vi "TCPServerListenLoop.vi"   [LabVIEW 2019]
uses:
  02 Mode/TCPServerMode/TCPServerClass.lvclass
types:
  T1 = typedef "队列枚举.ctl" = enum16{"ini", "读", "写"}
  T2 = map{string, refnum<class "TCPServerClass.lvclass">}
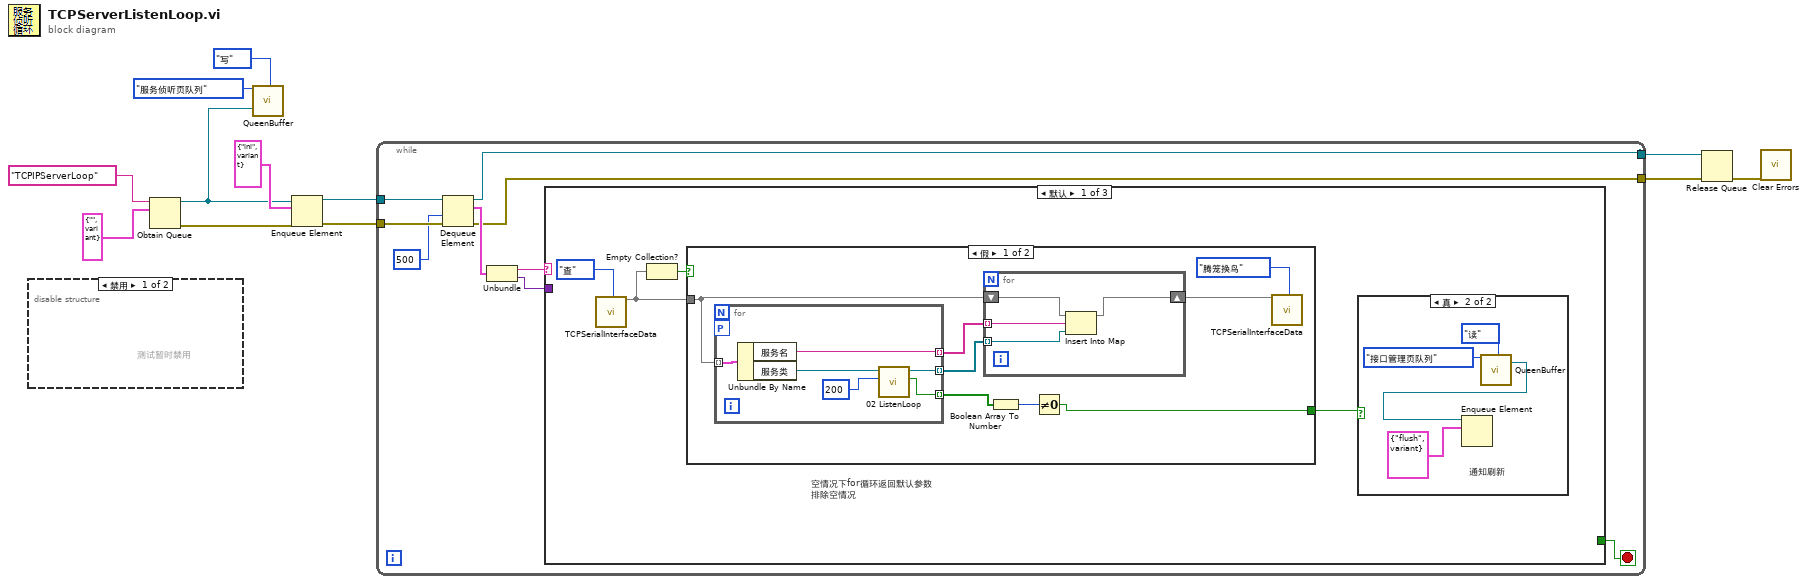
[diagram p0: block diagram]
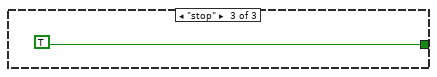
[diagram p6: hidden frame]
diagram:
  n1 = disable-structure shown="禁用" {
    frame Disabled {
      # "测试暂时禁用"
    }
    frame Enabled {
    }
  }
  n2 = Obtain Queue(name (unnamed)="TCPIPServerLoop" ("名称（未命名）"), element data type=cluster{string, variant} {"", variant}) -> (queue out=w1:refnum<queue>, error out=w4:errorcluster)  [unwired: 3 in, 1 out]
  n3 = call "QueenBuffer.vi"("名称"=enum16{"接口管理页队列", "服务侦听页队列", "主页队列"}."服务侦听页队列", "目标队列输入"=w1, "操作"=队列枚举."写") -> ()  [unwired: 16 in, 1 out]
  n4 = Enqueue Element(queue=w1, element=cluster{string, variant} {"ini", variant} ("元素"), error in (no error)=w4) -> (queue out=w11:refnum<queue>, error out=w10:errorcluster)  [unwired: 1 in, 1 out]
  n5 = while {
    tunnel: w11 -> [w21]
    tunnel: w10 -> [w20]
    tunnel: [w16] -> w9
    tunnel: [w15] -> w8
    stop <- w14 stop-if-true
    n6 = Dequeue Element(queue=w21, timeout in ms (-1)=500 ("超时毫秒(-1)"), error in (no error)=w20) -> (queue out=w16:refnum<queue>, element=w19:cluster{string, variant}, error out=w15:errorcluster)  [unwired: 1 out]
    n7 = Unbundle(w19) -> (w18:string, w17:variant)
    n8 = case shown="默认" w18 {
      tunnel: w17 -> [_ _ _]
      tunnel: [_ _ TRUE ("停止")] -> w14
      frame Default {
        # "空情况下for循环返回默认参数\n排除空情况"
        n9 = call "TCPSerialInterfaceData.vi"("客服接口枚举"=enum16{"ini", "增", "删", "查", "改"}."查") -> ("服务表"=w24:T2)  [unwired: 17 in, 1 out]
        n10 = Empty Collection?(1:w24) -> (0:w23:bool)
        n11 = case shown="假" w23 {
          tunnel: w24 -> [w33 _]
          tunnel: [w30 _] -> w22
          frame False {
            n12 = for {
              tunnel: w33 -> [w47] mode=indexing
              tunnel: [w44] -> w37 mode=indexing
              tunnel: [w43] -> w36 mode=indexing
              workers-P: _ -> [_]
              tunnel: [w42] -> w32 mode=indexing
              n13 = Unbundle By Name(w47) -> ("服务名"=w43:string, "服务类"=w46:refnum<class "TCPServerClass.lvclass">)
              n14 = call-dynamic "02 ListenLoop.vi"("超时毫秒"=200, "TCPServerClass 输入"=w46) -> ("新增"=w42:bool, "TCPServerClass 输出"=w44:refnum<class "TCPServerClass.lvclass">)  [unwired: 7 in, 1 out]
            }
            n15 = for {
              tunnel: w37 -> [w40] mode=indexing
              tunnel: w36 -> [w41] mode=indexing
              shift-right: [w38] -> w35
              shift-left: w33 -> [w39]
              n16 = Insert Into Map(map in=w39, key=w41, value=w40) -> (map out=w38:T2)  [unwired: 2 out]
            }
            n17 = Boolean Array To Number(Boolean array=w32) -> (number=w31:u32)
            n18 = Not Equal To 0?(x=w31) -> (x != 0?=w30:bool)
            n19 = call "TCPSerialInterfaceData.vi"("整体更新"=w35, "客服接口枚举"=enum16{"ini", "增", "删", "查", "改", "腾笼换鸟"}."腾笼换鸟") -> ()  [unwired: 16 in, 2 out]
          }
          frame True {
          }
        }
        n20 = case shown="真" w22 {
          frame False {
          }
          frame True {
            # "通知刷新"
            n21 = call "QueenBuffer.vi"("名称"=enum16{"接口管理页队列", "服务侦听页队列", "主页队列"}."接口管理页队列", "操作"=队列枚举."读") -> ("目标队列"=w29:refnum<queue>)  [unwired: 17 in]
            n22 = Enqueue Element(queue=w29, element=cluster{"字符串":string, variant} {"字符串"="flush", variant} ("元素")) -> ()  [unwired: 2 in, 3 out]
          }
        }
      }
      frame "ini" {
      }
      frame "stop" {
      }
    }
  }
  n23 = Release Queue(queue=w9, error in (no error)=w8) -> (error out=w7:errorcluster)  [unwired: 1 in, 2 out]
  n24 = call <vilib>:"Clear Errors.vi"("error in (no error)"=w7) -> ()  [unwired: 5 in, 2 out]
